vi "testtestteat.vi"() -> ()   [LabVIEW 2010]
panel:
  out "Numeric":dbl
  in  "Array":dbl[](array[numeric])
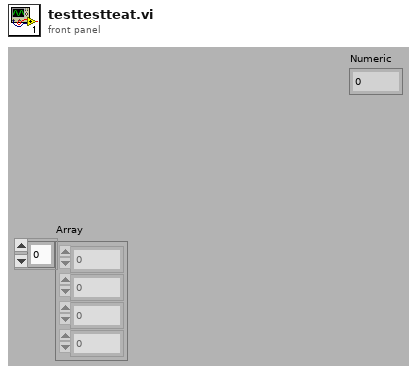
[diagram p1: front panel]
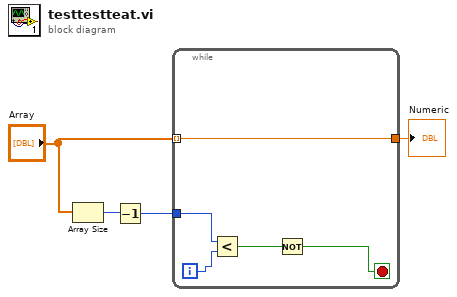
[diagram p0: block diagram]
diagram:
  n1 = Array Size(array="Array") -> (size(s)=w3:i32)
  n2 = Decrement(x=w3) -> (x-1=w2:i32)
  n3 = while {
    tunnel: "Array" -> [w6] mode=indexing
    tunnel: w2 -> [w9]
    tunnel: [w6] -> w1
    i -> [w8]
    stop <- w5 stop-if-true
    n4 = Less?(x=w9, y=w8) -> (x < y?=w7:bool)
    n5 = Not(x=w7) -> (.not. x?=w5:bool)
  }
  "Numeric" <- w1
